vi "Set-selected-motors.vi"(8 "error in (no error)":errorcluster, 10 "Active?":bool[](array[boolean]), 11 "Object ref in":T1) -> (0 "error out":errorcluster, 3 "Object ref out":T1)   [LabVIEW 2013, in "PowderDeposition.lvlib" / "PD-Main.lvclass"]
uses:
  PD-Main.lvclass
  Object-reference.ctl
  PD-Main.lvclass/PD-Main.ctl
  Read Motors-selection.vi
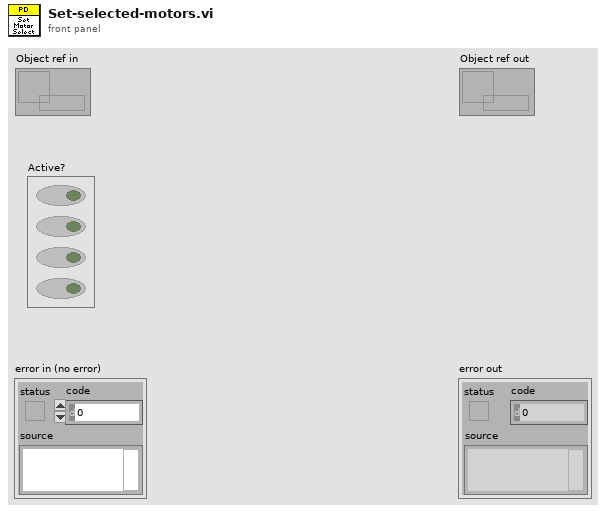
[diagram p1: front panel]
types:
  T1 = typedef "PowderDeposition.lvlib/PD-Main.lvclass/Object-reference.ctl" = refnum<data-value>
  T2 = cluster{"Active?[0]":bool, "Active?[1]":bool, "Active?[2]":bool, "Active?[3]":bool}
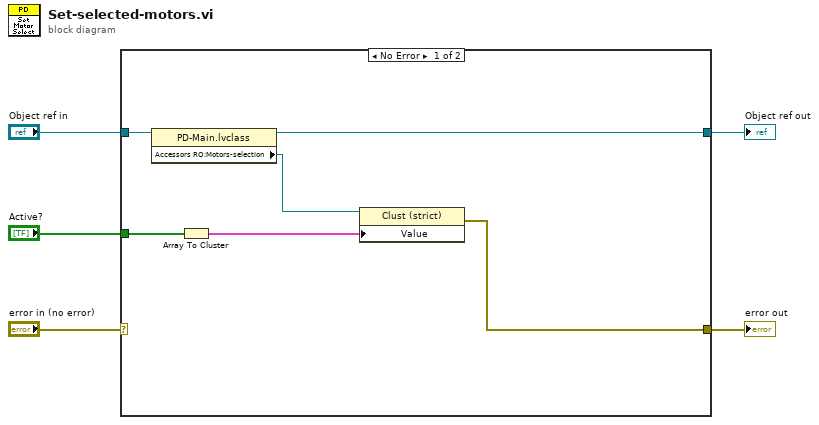
[diagram p0: block diagram]
diagram:
  n1 = case shown="No Error" "error in (no error)" {
    selector: "error in (no error)" -> [_ w13]
    tunnel: [w9 w13] -> w4
    tunnel: [w10 w12] -> w2
    tunnel: "Object ref in" -> [w11 w12]
    tunnel: "Active?" -> [w8 _]
    frame No Error {
      n2 = property class="PD-Main.lvclass"(reference=w11) -> (reference out=w10:T1, "Accessors RO:Motors-selection"=w7:refnum<vi>)  [unwired: 1 in, 1 out]
      n3 = Array To Cluster(array=w8) -> (cluster=w6:T2)
      n4 = property class="Clust (strict)"(reference=w7, "Value"=w6) -> (error out=w9:errorcluster)  [unwired: 1 in, 1 out]
    }
    frame Error {
    }
  }
  "error out" <- w4
  "Object ref out" <- w2
